vi "MeasCfg.vi"(0 "DigitsIn":i32=5 caption="No of Digits" min=3 max=6 step=1, 1 "TauIn":dbl=5.0 caption="Tau / s" min=0.1 max=30.0 step=0.1 format="%.1f", 3 "AvgIn":i32=100 caption="Averaging" min=1 max=999999 step=1, 4 "TrigIn":dbl=5.0 caption="Trigger Level" min=1.0 max=100.0 format="%_3f", 5 "DiaIn":dbl=5.0 caption="D" min=0.0 format="%_4f", 6 "AttIn":dbl caption="Attenuation" min=-60.0 max=60.0 step=1.0 format="%#.3f", 7 "Type":u16, 8 "VISA In":refnum<visa-resource-name>, 9 "Sensor?":bool, 10 "Adapter":enum32{"PD", "TH", "PY"}(radio), 11 "BWIn":u16(ring) caption="Bandwidth" items=["HIGH", "LOW"], 13 "Tau?":bool, 14 "ACCIn":string(combo)="AUTO" caption="Accelerator") -> (12 "Ini":bool, 15 "DiaSet":dbl, 16 "ACCOut":string, 17 "BWOut":u16(ring) items=["HIGH", "LOW"], 19 "AttOut":dbl caption="Attenuation" format="%_4f", 20 "DigitsOut":i32, 21 "AvgOut":i32=100, 23 "TauIOut":dbl=5.0 caption="Tau" format="%_4f", 24 "TrigOut":dbl=5.0 caption="Trig", 25 "DiaOut":dbl=5.0 caption="Beam Dia", 27 "AOutcm²":dbl=5.0)   [LabVIEW 2015]
panel:
  out "AdapterOut":enum32{"PD", "TH", "PY"}(radio)
  out "Zero":dbl format="%#_4p"
  in  "DiaIn 2":dbl=5.0 caption="Y" format="%_4f"
  in  "Beam Setup":T1(radio)
  in  "Zero":bool
  in  "stop":bool
  # "Configure Measurement"
  # "Pyro:\n- Trigger"
  # "General\n- Beam Dia\n- Zero Adj"
  # "Thermo:\n- Accelerator"
  # "Photo:\n- Bandwidth"
  # "- No of Digits\n- Averaging Rate"
  # "dB"
  # "mm"
  # "mm"
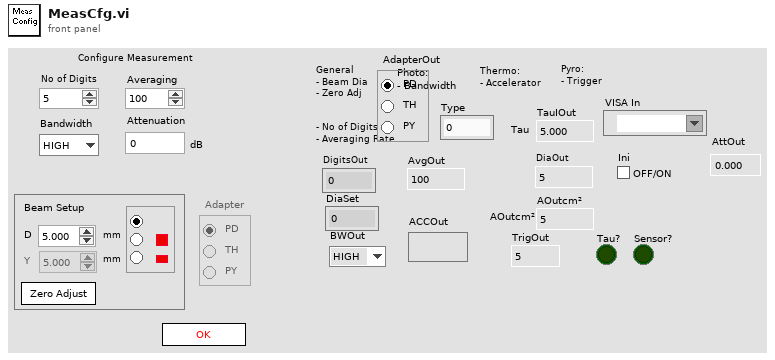
[diagram p1: front panel]
types:
  T1 = enum32{"Radio Selection 1", "Radio Selection 2", "Radio Selection 3"}
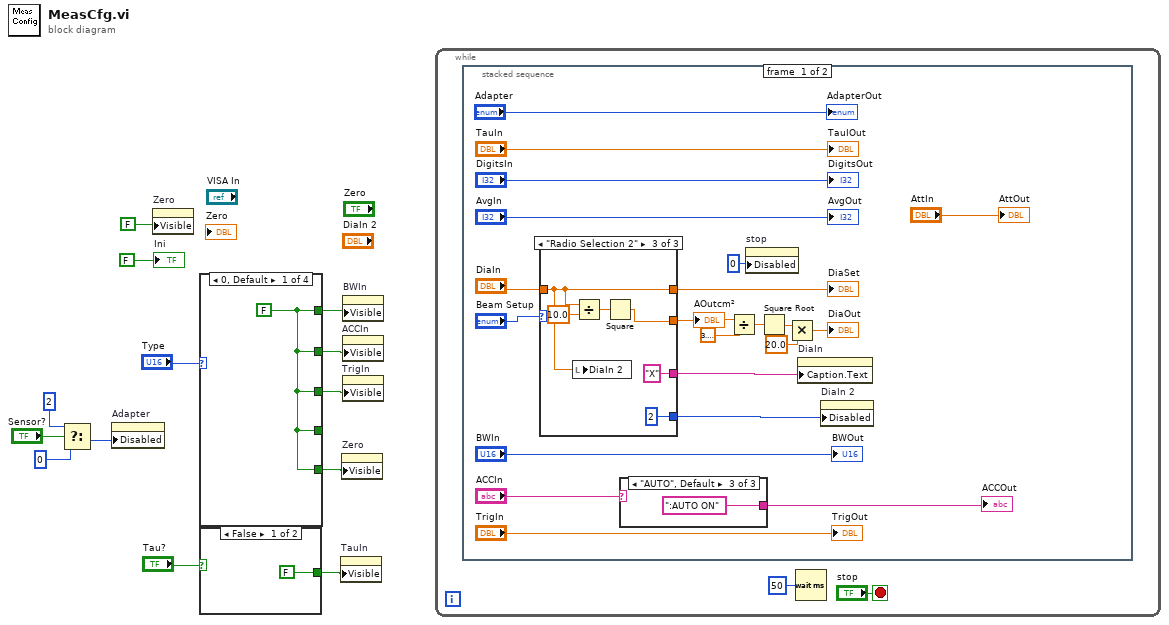
[diagram p0: block diagram]
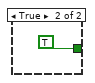
[diagram p2: hidden frame]
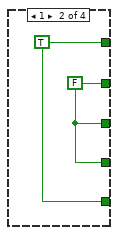
[diagram p3: hidden frame]
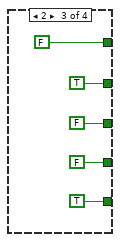
[diagram p4: hidden frame]
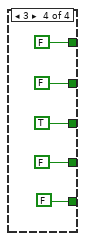
[diagram p5: hidden frame]
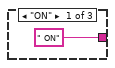
[diagram p6: hidden frame]
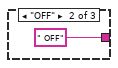
[diagram p7: hidden frame]
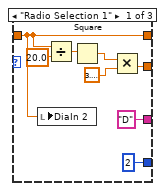
[diagram p8: hidden frame]
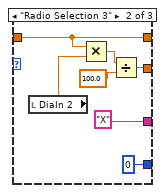
[diagram p9: hidden frame]
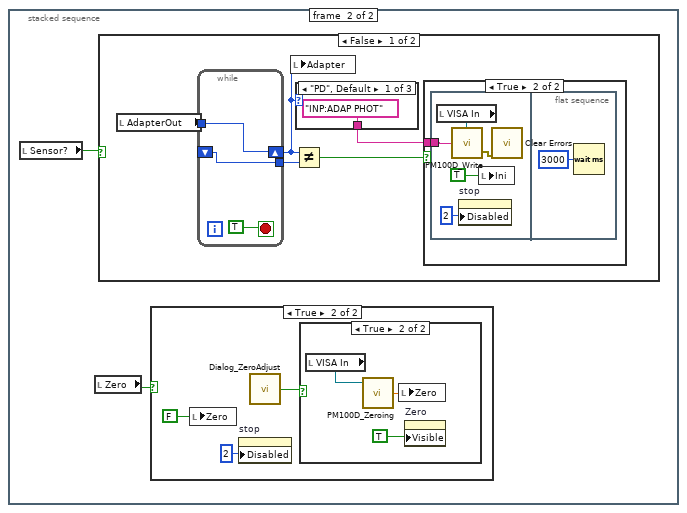
[diagram p10: hidden frame]
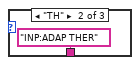
[diagram p11: hidden frame]
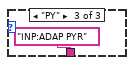
[diagram p12: hidden frame]
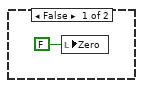
[diagram p15: hidden frame]
diagram:
  n1 = Select(t=2, s="Sensor?", f=0) -> (s? t:f=w3:i32)
  n2 = property on="Adapter" class="RadioBtnsControl (strict)"("Disabled"=w3) -> ()  [unwired: 2 in, 2 out]
  n3 = property on="Zero" class="DigNum (strict)"("Visible"=FALSE) -> ()  [unwired: 2 in, 2 out]
  n4 = case shown="0, Default" "Type" {
    tunnel: [w14 w15 FALSE FALSE] -> w12
    tunnel: [w14 w16 TRUE FALSE] -> w11
    tunnel: [w14 w16 FALSE TRUE] -> w10
    tunnel: [w14 w16 FALSE FALSE] -> _
    tunnel: [w14 w15 TRUE FALSE] -> w9
    frame 0, Default {
      w14 = FALSE
    }
    frame 1 {
      w16 = FALSE
      w15 = TRUE
    }
    frame 2 {
    }
    frame 3 {
    }
  }
  n5 = case shown="False" "Tau?" {
    tunnel: [FALSE TRUE] -> w7
    frame False {
    }
    frame True {
    }
  }
  n6 = property on="TauIn" class="DigNum (strict)"("Visible"=w7) -> ()  [unwired: 2 in, 2 out]
  n7 = property on="Zero" class="Bool (strict)"("Visible"=w9) -> ()  [unwired: 2 in, 2 out]
  n8 = property on="BWIn" class="Ring (strict)"("Visible"=w12) -> ()  [unwired: 2 in, 2 out]
  n9 = property on="ACCIn" class="CmbBox"("Visible"=w11) -> ()  [unwired: 2 in, 2 out]
  n10 = property on="TrigIn" class="DigNum (strict)"("Visible"=w10) -> ()  [unwired: 2 in, 2 out]
  n11 = while {
    stop <- "stop" stop-if-true
    n12 = stacked-sequence {
      frame #0 {
        n13 = case shown="\"Radio Selection 2\"" "Beam Setup" {
          tunnel: [w56 w68 w71] -> w38
          tunnel: "DiaIn" -> [w56 w68 w71]
          tunnel: [w58 w66 w73] -> w45
          tunnel: ["D" "X" "X"] -> w48
          tunnel: [2 0 2] -> w47
          frame "Radio Selection 1" {
            n14 = local write "DiaIn 2"(w56) -> ()
            n15 = Divide(x=w56, y=20.0) -> (x/y=w61:dbl)
            n16 = Square(x=w61) -> (x^2=w60:dbl)
            n17 = Multiply(x=w60, y=3.141592653589793) -> (x*y=w58:dbl)
          }
          frame "Radio Selection 3" {
            n18 = local read "DiaIn 2"() -> (w64:dbl)
            n19 = Multiply(x=w68, y=w64) -> (x*y=w67:dbl)
            n20 = Divide(x=w67, y=100.0) -> (x/y=w66:dbl)
          }
          frame "Radio Selection 2" {
            n21 = local write "DiaIn 2"(w71) -> ()
            n22 = Divide(x=w71, y=10.0) -> (x/y=w74:dbl)
            n23 = Square(x=w74) -> (x^2=w73:dbl)
          }
        }
        "AOutcm²" <- w45
        "DiaSet" <- w38
        n24 = case shown="\"AUTO\", Default" "ACCIn" {
          tunnel: [" ON" ("ACCOut") " OFF" ("ACCOut") ":AUTO ON" ("ACCOut")] -> w32
          frame "ON" {
          }
          frame "OFF" {
          }
          frame "AUTO", Default {
          }
        }
        "ACCOut" <- w32
        n25 = Divide(x=w45, y=3.141592653589793) -> (x/y=w43:dbl)
        n26 = property on="stop" class="Bool"("Disabled"=u8 0) -> ()  [unwired: 2 in, 2 out]
        n27 = Square Root(x=w43) -> (sqrt(x)=w42:dbl)
        n28 = Multiply(x=w42, y=20.0) -> (x*y=→"DiaOut":dbl)
        n29 = property on="DiaIn" class="DigNum (strict)"("Caption.Text"=w48) -> ()  [unwired: 2 in, 2 out]
        n30 = property on="DiaIn 2" class="DigNum (strict)"("Disabled"=w47) -> ()  [unwired: 2 in, 2 out]
        "DigitsOut" <- "DigitsIn"
        "AvgOut" <- "AvgIn"
        "TrigOut" <- "TrigIn"
        "BWOut" <- "BWIn"
        "TauIOut" <- "TauIn"
        "AdapterOut" <- "Adapter"
        "AttOut" <- "AttIn"
      }
      frame #1 {
        n31 = local read "Sensor?"() -> (w76:bool)
        n32 = local read "Zero"() -> (w77:bool)
        n33 = case shown="False" w76 {
          frame False {
            n34 = local read "AdapterOut"() -> (w79:enum32{"PD", "TH", "PY"})
            n35 = while {
              shift-right: [w94] -> w78
              shift-left: _ -> [w93]
              tunnel: w79 -> [w94]
              tunnel: [w93] -> w82
              stop <- TRUE stop-if-true
            }
            n36 = local write "Adapter"(w78) -> ()
            n37 = Not Equal?(x=w78, y=w82) -> (x != y?=w81:bool)
            n38 = case shown="\"PD\", Default" w78 {
              tunnel: ["INP:ADAP PHOT" "INP:ADAP THER" "INP:ADAP PYR"] -> w80
              frame "PD", Default {
              }
              frame "TH" {
              }
              frame "PY" {
              }
            }
            n39 = case shown="True" w81 {
              tunnel: w80 -> [_ w86]
              frame False {
              }
              frame True {
                n40 = flat-sequence {
                  tunnel: w86 -> [w90]
                  frame #0 {
                    n41 = local read "VISA In"() -> (w91:refnum<visa-resource-name>)
                    n42 = call "PM100D_Write.vi"("Command"=w90, "VISA in"=w91) -> ("error out"=w87:errorcluster)  [unwired: 1 in, 1 out]
                    n43 = property on="stop" class="Bool"("Disabled"=u8 2) -> ()  [unwired: 2 in, 2 out]
                    n44 = local write "Ini"(TRUE ("Ini")) -> ()
                    n45 = call <vilib>:"Clear Errors.vi"("error in (no error)"=w87) -> ()  [unwired: 5 in, 2 out]
                  }
                  frame #1 {
                    n46 = Wait (ms)(milliseconds to wait=u32 3000) -> ()  [unwired: 1 out]
                  }
                }
              }
            }
          }
          frame True {
          }
        }
        n47 = case shown="True" w77 {
          frame False {
            n48 = local write "Zero"(FALSE ("Zero")) -> ()
          }
          frame True {
            n49 = local write "Zero"(FALSE ("Zero")) -> ()
            n50 = property on="stop" class="Bool"("Disabled"=u8 2) -> ()  [unwired: 2 in, 2 out]
            n51 = call "Dialog_ZeroAdjust.vi"() -> ("OK"=w97:bool)  [unwired: 7 in]
            n52 = case shown="True" w97 {
              frame False {
              }
              frame True {
                n53 = local read "VISA In"() -> (w102:refnum<visa-resource-name>)
                n54 = call "PM100D_Zeroing.vi"("VISA In"=w102) -> ("ZeroValue"=w101:dbl)  [unwired: 4 in]
                n55 = local write "Zero"(w101) -> ()
                n56 = property on="Zero" class="DigNum (strict)"("Visible"=TRUE) -> ()  [unwired: 2 in, 2 out]
              }
            }
          }
        }
      }
    }
    n57 = Wait (ms)(milliseconds to wait=u32 50) -> ()  [unwired: 1 out]
  }
  "Ini" <- FALSE ("Ini")
